vi "TIO Avg Data.vi"(2 "Tableau":T2(array[cluster]), 8 "entrée d'erreur (pas d'erreur)":errorcluster) -> (0 "sortie d'erreur":errorcluster)   [LabVIEW 2010]
panel:
  out "élément":T1
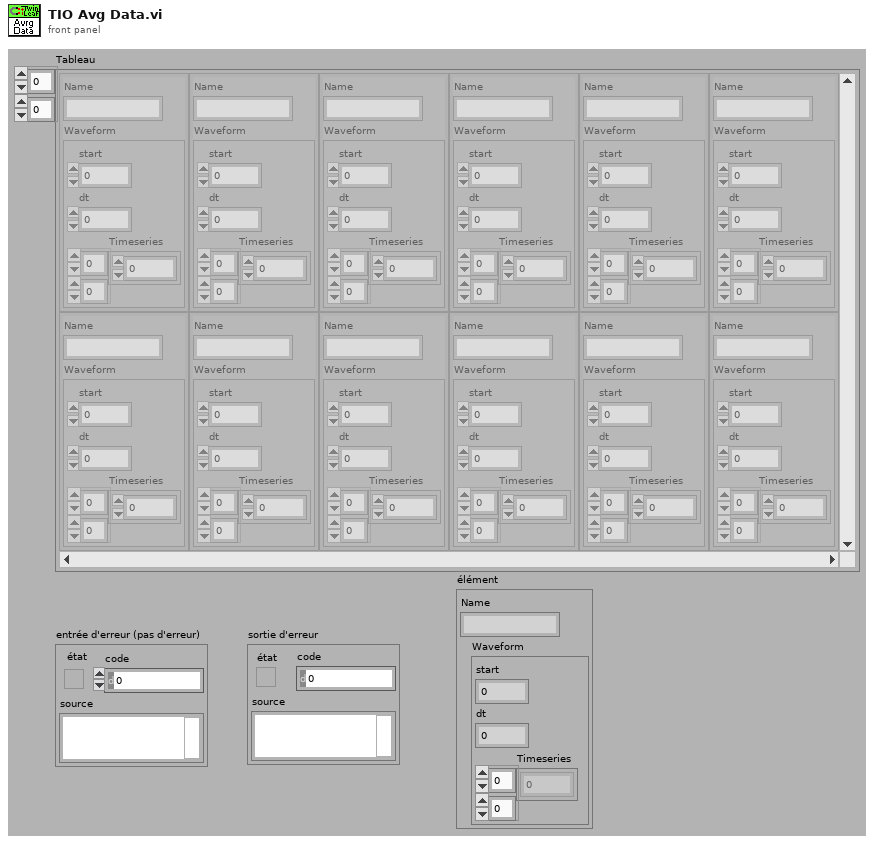
[diagram p1: front panel]
types:
  T1 = cluster{"Name":string, "Waveform":cluster{"start":dbl, "dt":dbl, "Timeseries":dbl[][]}}
  T2 = cluster{"Name":string, "Waveform":cluster{"start":dbl, "dt":dbl, "Timeseries":dbl[][]}}[][]
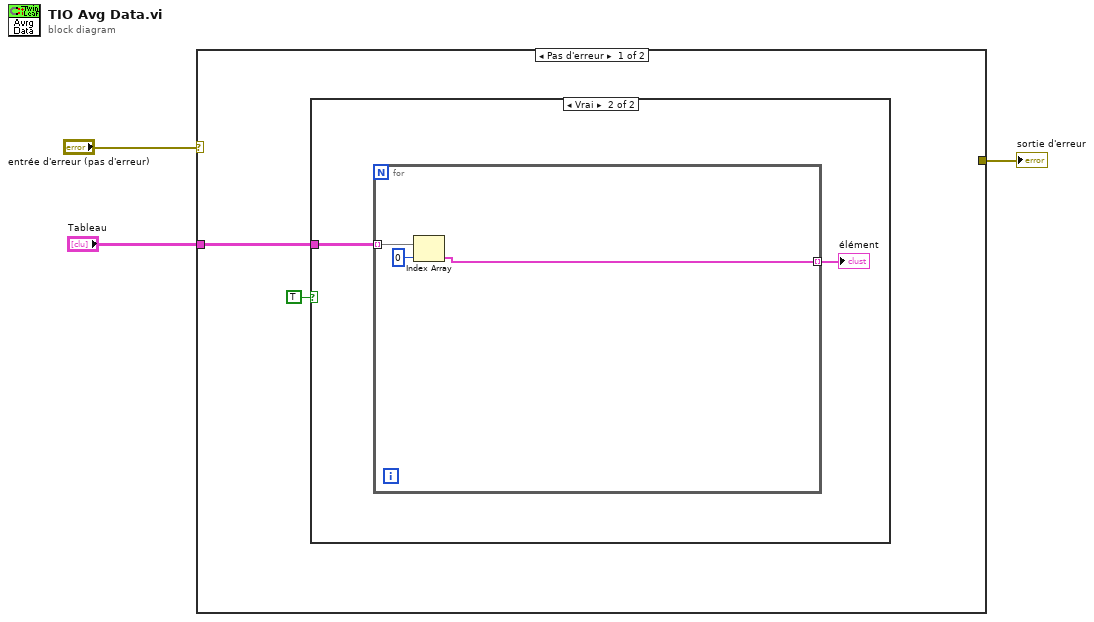
[diagram p0: block diagram]
diagram:
  n1 = case shown="Pas d'erreur" "entrée d'erreur (pas d'erreur)" {
    selector: "entrée d'erreur (pas d'erreur)" -> [_ w11]
    tunnel: [_ w11] -> w2
    tunnel: "Tableau" -> [w5 _]
    frame No Error {
      n2 = case shown="Vrai" TRUE {
        tunnel: w5 -> [_ w7]
        frame False {
        }
        frame True {
          n3 = for {
            tunnel: w7 -> [w10] mode=indexing
            tunnel: [w8] -> w6 mode=indexing
            n4 = Index Array(array=w10, index=0 ("indice")) -> (element=w8:T1)
          }
          "élément" <- w6
        }
      }
    }
    frame Error {
    }
  }
  "sortie d'erreur" <- w2
